vi "Test Basic Operations 2.vi"() -> ()   [LabVIEW 2014]
uses:
  <vilib>/Aledyne-TSXperts/Arduino Compatible Compiler for LabVIEW/Arduino Compatible Compiler for LabVIEW.lvlib
  <vilib>/Aledyne-TSXperts/Arduino Compatible Compiler for LabVIEW/addons/Complex Numbers/Complex Numbers.lvlib
panel:
  out "error out":errorcluster
  in  "error in (no error)":errorcluster
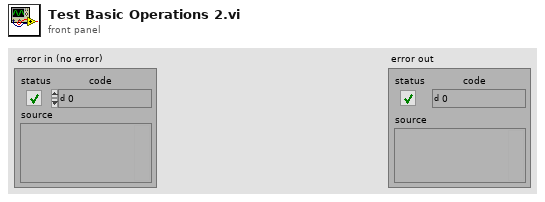
[diagram p1: front panel]
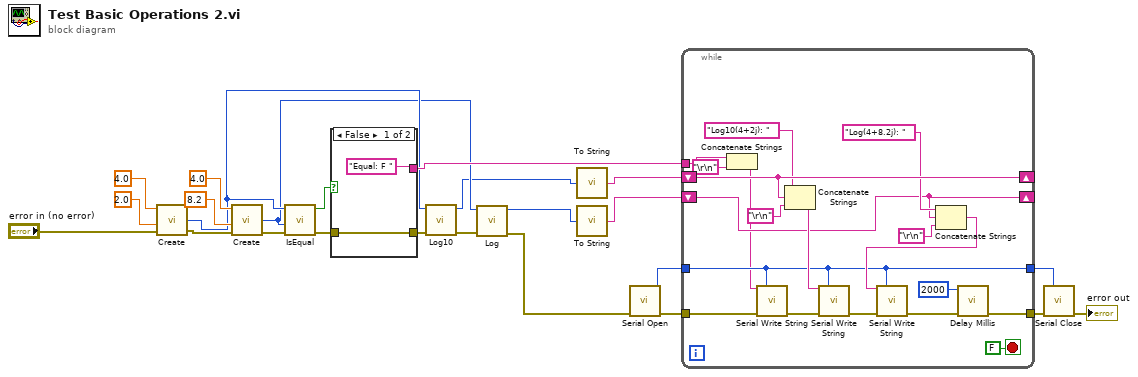
[diagram p0: block diagram]
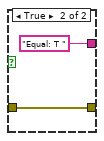
[diagram p2: hidden frame]
diagram:
  n1 = call <vilib>:"Create.vi"("Error In"="error in (no error)", "Imag"=2.0, "Real"=4.0) -> ("Error Out"=w9:errorcluster, "Complex"=w4:u32)  [unwired: 2 in]
  n2 = call <vilib>:"Create.vi"("Error In"=w9, "Imag"=8.2, "Real"=4.0) -> ("Error Out"=w10:errorcluster, "Complex"=w3:u32)  [unwired: 2 in]
  n3 = call <vilib>:"IsEqual.vi"("Error In"=w10, "B"=w3, "A"=w4) -> ("Error Out"=w7:errorcluster, "Equal?"=w6:bool)  [unwired: 7 in]
  n4 = case shown="False" w6 {
    tunnel: [w26 w28] -> w8
    tunnel: w7 -> [w26 w28]
    tunnel: ["Equal: F " ("string") "Equal: T " ("string")] -> w5
    frame False {
    }
    frame True {
    }
  }
  n5 = call <vilib>:"Log10.vi"("Error In"=w8, "A"=w4) -> ("Error Out"=w14:errorcluster, "log10(A)"=w2:u32)  [unwired: 8 in]
  n6 = call <vilib>:"Log.vi"("Error In"=w14, "A"=w3) -> ("Error Out"=w13:errorcluster, "log(A)"=w1:u32)  [unwired: 8 in]
  n7 = call <vilib>:"To String.vi"("Complex number"=w2) -> ("String complex num."=w15:string)
  n8 = call <vilib>:"To String.vi"("Complex number"=w1) -> ("String complex num."=w16:string)
  n9 = call <vilib>:"Serial Open.vi"("error in (no error)"=w13) -> ("Instance"=w22:u8, "error out"=w24:errorcluster)  [unwired: 13 in]
  n10 = while {
    tunnel: w24 -> [w34]
    tunnel: [w45] -> w23
    tunnel: w22 -> [w33]
    tunnel: [w33] -> w21
    shift-right: [w38] -> _
    shift-left: w15 -> [w38]
    shift-right: [w36] -> _
    shift-left: w16 -> [w36]
    tunnel: w5 -> [w31]
    stop <- FALSE stop-if-true
    n11 = Concatenate Strings(w31, "\r\n") -> (w29:string)
    n12 = call <vilib>:"Serial Write String.vi"("String"=w29, "Instance"=w33, "error in (no error)"=w34) -> ("error out"=w35:errorcluster)  [unwired: 12 in]
    n13 = Concatenate Strings("Log10(4+2j): " ("string"), w38, "\r\n") -> (w40:string)
    n14 = call <vilib>:"Serial Write String.vi"("String"=w40, "Instance"=w33, "error in (no error)"=w35) -> ("error out"=w43:errorcluster)  [unwired: 12 in]
    n15 = Concatenate Strings("Log(4+8.2j): " ("string"), w36, "\r\n") -> (w39:string)
    n16 = call <vilib>:"Serial Write String.vi"("String"=w39, "Instance"=w33, "error in (no error)"=w43) -> ("error out"=w46:errorcluster)  [unwired: 12 in]
    n17 = call <vilib>:"Delay Millis.vi"("error in (no error)"=w46, "delay"=u32 2000) -> ("error out"=w45:errorcluster)  [unwired: 9 in]
  }
  n18 = call <vilib>:"Serial Close.vi"("Instance"=w21, "error in (no error)"=w23) -> ("error out"=→"error out":errorcluster)  [unwired: 13 in]
